vi "roboRIO v1.0 CAN Interface Manager.vi"(7 "Action":T1, 8 "error in (no error)":errorcluster, 11 "CAN Interface Obj in":refnum<k20>) -> (0 "error out":errorcluster, 3 "CAN Interface Obj out":refnum<k20>)   [LabVIEW 2021]
uses:
  <vilib>/myRIO/Common/Instrument Driver Framework/Utilities/typedefs/FPGA Ref Manager Action Enum.ctl
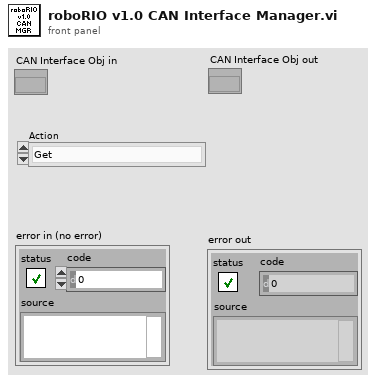
[diagram p1: front panel]
types:
  T1 = typedef "FPGA Ref Manager Action Enum.ctl" = enum16{"Get", "Set", "Reset"}
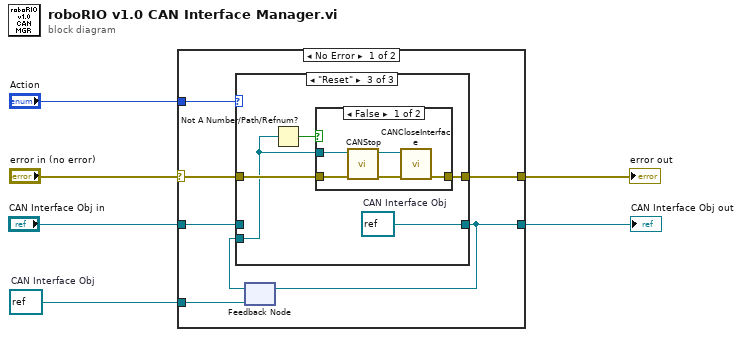
[diagram p0: block diagram]
diagram:
  w3 = refnum<k20> refnum  # CAN Interface Obj
  n1 = case shown="No Error" "error in (no error)" {
    selector: "error in (no error)" -> [w9 w29]
    tunnel: "Action" -> [w12 _]
    tunnel: w3 -> [w11 w30]
    tunnel: [w10 w29] -> w5
    tunnel: [w8 w30] -> w2
    tunnel: "CAN Interface Obj in" -> [w7 _]
    frame No Error {
      n2 = feedback #1(w11) -> (w13:refnum<k20>)
      n3 = case shown="\"Reset\"" w12 {
        tunnel: [w14 w16 w22] -> w8
        tunnel: w13 -> [_ w16 w18]
        tunnel: w9 -> [w15 w17 w20]
        tunnel: [w15 w17 w21] -> w10
        tunnel: w7 -> [w14 _ _]
        frame "Set" {
        }
        frame "Get" {
        }
        frame "Reset" {
          w22 = refnum<k20> refnum  # CAN Interface Obj
          n4 = Not A Number/Path/Refnum?(number/path/refnum=w18) -> (NaN/Path/Refnum?=w19:bool)
          n5 = case shown="False" w19 {
            tunnel: [w27 w28] -> w21
            tunnel: w20 -> [w26 w28]
            tunnel: w18 -> [w23 _]
            frame False {
              n6 = call <vilib>:"CANStop.vi"("error in (no error)"=w26, "interface object in"=w23) -> ("error out"=w25:errorcluster, "interface object out"=w24:refnum<k20>)  [unwired: 8 in]
              n7 = call <vilib>:"CANCloseInterface.vi"("error in (no error)"=w25, "interface object in"=w24) -> ("error out"=w27:errorcluster)  [unwired: 9 in]
            }
            frame True {
            }
          }
        }
      }
      n8 = feedback-in #1(w8) -> ()
    }
    frame Error {
    }
  }
  "error out" <- w5
  "CAN Interface Obj out" <- w2
